vi "Get I Am.vi"(8 "error in (no error)":errorcluster, 11 "niDTS BT DUT in":refnum<class "niDTS BT Dut.lvclass">) -> (0 "error out":errorcluster, 2 "I Am":string, 3 "niDTS BT DUT out":refnum<class "niDTS BT Dut.lvclass">)   [LabVIEW 2015, in "niDTS BT.lvlib" / "niDTS BT Dut.lvclass"]
uses:
  niDTS BT Dut.lvclass
panel:
  # "This is used for testing the dispatching of the plugins"
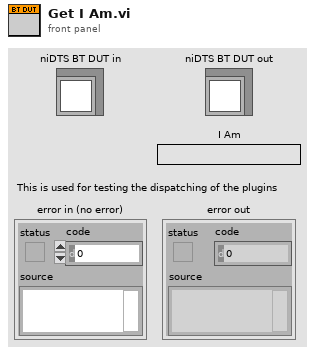
[diagram p1: front panel]
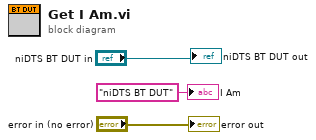
[diagram p0: block diagram]
diagram:
  "error out" <- "error in (no error)"
  "niDTS BT DUT out" <- "niDTS BT DUT in"
  "I Am" <- "niDTS BT DUT" ("I Am")
